vi "Set Size.vi"(8 "error in (no error)":errorcluster, 10 "Size":i32, 11 "Map in":refnum<class "Map.lvclass">) -> (0 "error out":errorcluster, 3 "Map out":refnum<class "Map.lvclass">)   [LabVIEW 2020, in "SquareBattle.lvlib" / "Map.lvclass"]
uses:
  Map.lvclass
  Square/Square.lvclass
  Run Result.ctl
  Action.ctl
  Direction.ctl
  Map.lvclass/Map.ctl
  SquareBattle.lvlib
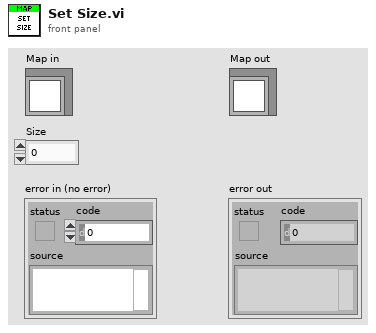
[diagram p1: front panel]
types:
  T1 = typedef "SquareBattle.lvlib/Run Result.ctl" = cluster{"Action":T2, "Direction":T3, "Replication":refnum<class "Square.lvclass">}
  T2 = typedef "SquareBattle.lvlib/Action.ctl" = enum16{"Wait", "Move", "Attack", "Replicate"}
  T3 = typedef "SquareBattle.lvlib/Direction.ctl" = enum16{"NW", "N", "NE", "E", "SE", "S", "SW", "W"}
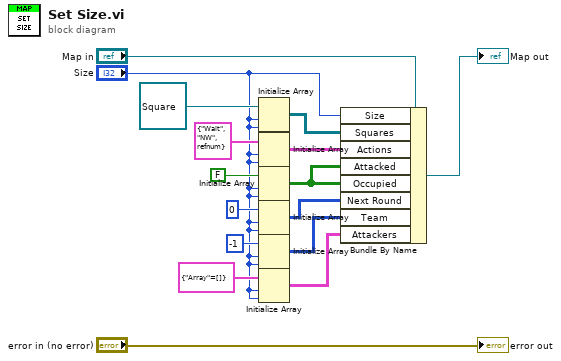
[diagram p0: block diagram]
diagram:
  n1 = Initialize Array(refnum<class "Square.lvclass"> refnum ("SquareBattle:Square"), "Size", "Size") -> (w5:refnum<class "Square.lvclass">[][])
  n2 = Initialize Array(T1 {"Action"=enum."Wait", "Direction"=enum."NW", "Replication"=refnum} ("Run Result"), "Size", "Size") -> (w14:T1[][])
  n3 = Initialize Array(FALSE, "Size", "Size") -> (w8:bool[][])
  n4 = Initialize Array(u32 0, "Size", "Size") -> (w10:u32[][])
  n5 = Initialize Array(-1, "Size", "Size") -> (w4:i32[][])
  n6 = Initialize Array(cluster{"Array":i32[]} {"Array"=[]} ("Attackers"), "Size", "Size") -> (w1:cluster{"Array":i32[]}[][])
  n7 = Bundle By Name(cluster="Map in", "Size"="Size", "Squares"=w5, "Actions"=w14, "Attacked"=w8, "Occupied"=w8, "Next Round"=w10, "Team"=w4, "Attackers"=w1) -> (→"Map out":refnum<class "Map.lvclass">)
  "error out" <- "error in (no error)"
